vi "Make Icons.vi"(10 "Display Name":string, 11 "palette config in":T1={"display name"="Lua", "view format"=0, "palette width"=2, "items"=[], "256 color icon"=bytes[1182], "B&W color icon"=bytes[286], "help information"={"help tag"="", "help file path "=path ""}, "palette description"="", "synchronize information"={"synchronize with directory"=FALSE, "synchronize directory path"=path ""}} {"view format" items=["Icons", "Text", "Icons and Text"]}) -> (3 "palette config out":T1={"display name"="Lua", "view format"=0, "palette width"=2, "items"=[], "256 color icon"=bytes[1182], "B&W color icon"=bytes[286], "help information"={"help tag"="", "help file path "=path ""}, "palette description"="", "synchronize information"={"synchronize with directory"=FALSE, "synchronize directory path"=path ""}} {"view format" items=["Icons", "Text", "Icons and Text"]})   [LabVIEW 2020, in "Lua DevUtil.lvlib"]
uses:
  Lua DevUtil.lvlib
  <vilib>/Palette API/Palette Menu/Public Type Define/Palette Data.ctl
  <vilib>/Palette API/Palette Menu/Public Type Define/View Format.ctl
  <vilib>/Palette API/Palette Menu/Public Type Define/Items.ctl
  <vilib>/Palette API/Palette Menu/Public Type Define/Item.ctl
  <vilib>/Palette API/Palette Menu/Public Type Define/Help Info.ctl
  <vilib>/Palette API/Palette Menu/Public Type Define/Synchronize Info.ctl
  <vilib>/Palette API/Palette Menu/Palette Menu.lvlib
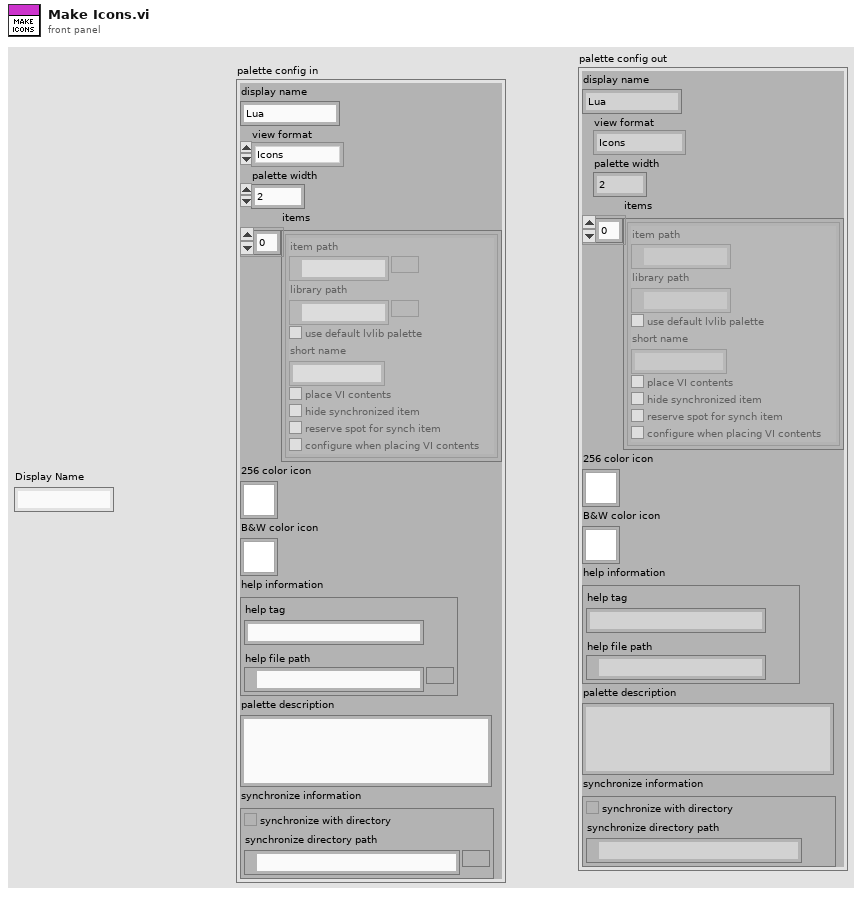
[diagram p1: front panel]
types:
  T1 = typedef "Palette Menu.lvlib/Palette Data.ctl" = cluster{"display name":string, "view format":T2, "palette width":i16, "items":T3, "256 color icon":picture, "B&W color icon":picture, "help information":T5, "palette description":string, "synchronize information":T6}
  T2 = typedef "Palette Menu.lvlib/View Format.ctl" = u16
  T3 = typedef "Palette Menu.lvlib/Items.ctl" = T4[]
  T4 = typedef "Palette Menu.lvlib/Item.ctl" = cluster{"item path":path, "library path":path, "use default lvlib palette":bool, "short name":string, "place VI contents":bool, "hide synchronized item":bool, "reserve spot for synch item":bool, "configure when placing VI contents":bool}
  T5 = typedef "Palette Menu.lvlib/Help Info.ctl" = cluster{"help tag":string, "help file path ":path}
  T6 = typedef "Palette Menu.lvlib/Synchronize Info.ctl" = cluster{"synchronize with directory":bool, "synchronize directory path":path}
  T7 = enum16{"User-specified Font", "Application Font", "System Font", "Dialog Font"}
  T8 = cluster{"Font Name:":string, "Size":i16, "Strikeout?":bool, "Italic?":bool, "Underline?":bool, "Outline?":bool, "Shadow?":bool, "Bold?":bool}
  T9 = cluster{"horizontal":enum16{"left", "center", "right"}, "vertical":enum16{"top", "center", "bottom"}}
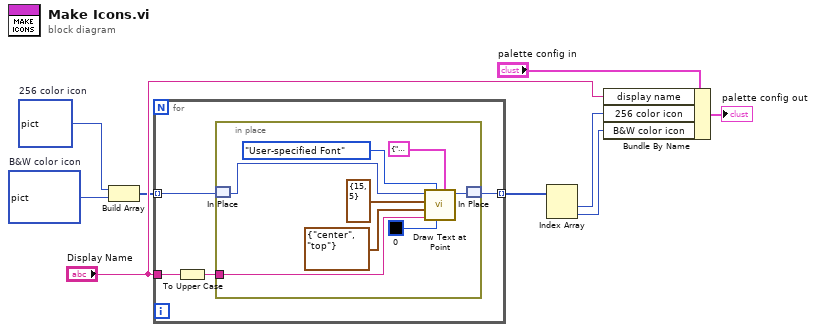
[diagram p0: block diagram]
diagram:
  w6 = picture bytes[1182]  # 256 color icon
  w5 = picture bytes[286]  # B&W color icon
  n1 = Build Array(w6, w5) -> (w4:picture[])
  n2 = for {
    tunnel: "Display Name" -> [w13]
    tunnel: w4 -> [w12] mode=indexing
    tunnel: [w11] -> w3 mode=indexing
    n3 = To Upper Case(1:w13) -> (0:w10:string)
    n4 = in-place {
      in-place-border: w10 -> [w14]
      n5 = in-place-match #1(w12) -> (w16:picture)
      n6 = call <vilib>:"Draw Text at Point.vi"("[user-specified font]"=T8 {"Font Name:"="Small Fonts", "Size"=9, "Strikeout?"=FALSE, "Italic?"=FALSE, "Underline?"=FALSE, "Outline?"=FALSE, "Shadow?"=FALSE, "Bold?"=FALSE}, "text color(black)"=u32 0, "desired font(Application)"=T7."User-specified Font", "text"=w14, "alignment(left, top)"=T9 {"horizontal"=enum."center", "vertical"=enum."top"}, "origin"=cluster{"x":i16, "y":i16} {"x"=15, "y"=5}, "picture"=w16) -> ("new picture"=w17:picture)  [unwired: 3 in, 1 out]
      n7 = in-place-match #1(w17) -> (w11:picture)
    }
  }
  n8 = Index Array(array=w3) -> (element #1=w2:picture, element #2=w1:picture)  [unwired: 2 in]
  n9 = Bundle By Name(cluster="palette config in", "display name"="Display Name", "256 color icon"=w2, "B&W color icon"=w1) -> (→"palette config out":T1)
